vi "6.vi"() -> ()   [LabVIEW 2017]
panel:
  out "字符串":string
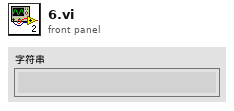
[diagram p1: front panel]
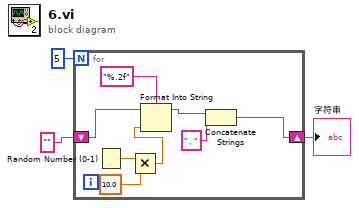
[diagram p0: block diagram]
diagram:
  n1 = for {
    N: 5 -> [_]
    shift-right: [w4] -> w1
    shift-left: "" -> [w10]
    n2 = Random Number (0-1)() -> (number: 0 to 1=w7:dbl)
    n3 = Multiply(x=w7, y=10.0) -> (x*y=w5:dbl)
    n4 = Format Into String(format string="%.2f" ("格式字符串"), initial string=w10, w5) -> (resulting string=w8:string)  [unwired: 1 in, 1 out]
    n5 = Concatenate Strings(w8, "，" ("字符串")) -> (w4:string)
  }
  "字符串" <- w1
